vi "frontEnd.vi"(8 "error in (no error)":errorcluster, 11 "PixelflySettings in":refnum<class "PixelflySettings.lvclass">) -> (0 "error out":errorcluster, 3 "PixelflySettings out":refnum<class "PixelflySettings.lvclass">)   [LabVIEW 2009, in "Tools.lvlib" / "Settings.lvlib" / "PixelflySettings.lvclass"]
uses:
  PixelflySettings.lvclass
  PixelflySettings.lvclass/PixelflySettings.ctl
panel:
  out "Path":path
  in  "Mode":enum16{"Asynch Shutter", "Video"}(ring)=enum."Video"
  in  "Vertical Binning":enum16{"1", "2"}(ring)
  in  "Horizonatal Binning":enum16{"1", "2"}(ring)
  in  "image_number":i32 caption="Image Number"
  in  "Close":bool
  in  "Open":bool
  in  "Save":bool
  in  "Triggering":bool
  in  "gain":enum16{"Low", "High"}(ring) caption="Gain"
  in  "exposure":dbl(slide)=0.0064 min=1e-05 max=10.0 step=1e-05 scale=0.01..10.0 scale format="%^#_6g"
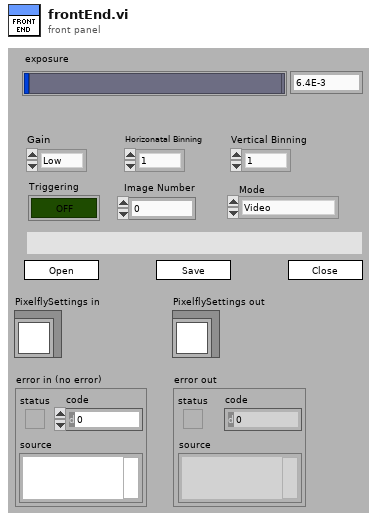
[diagram p1: front panel]
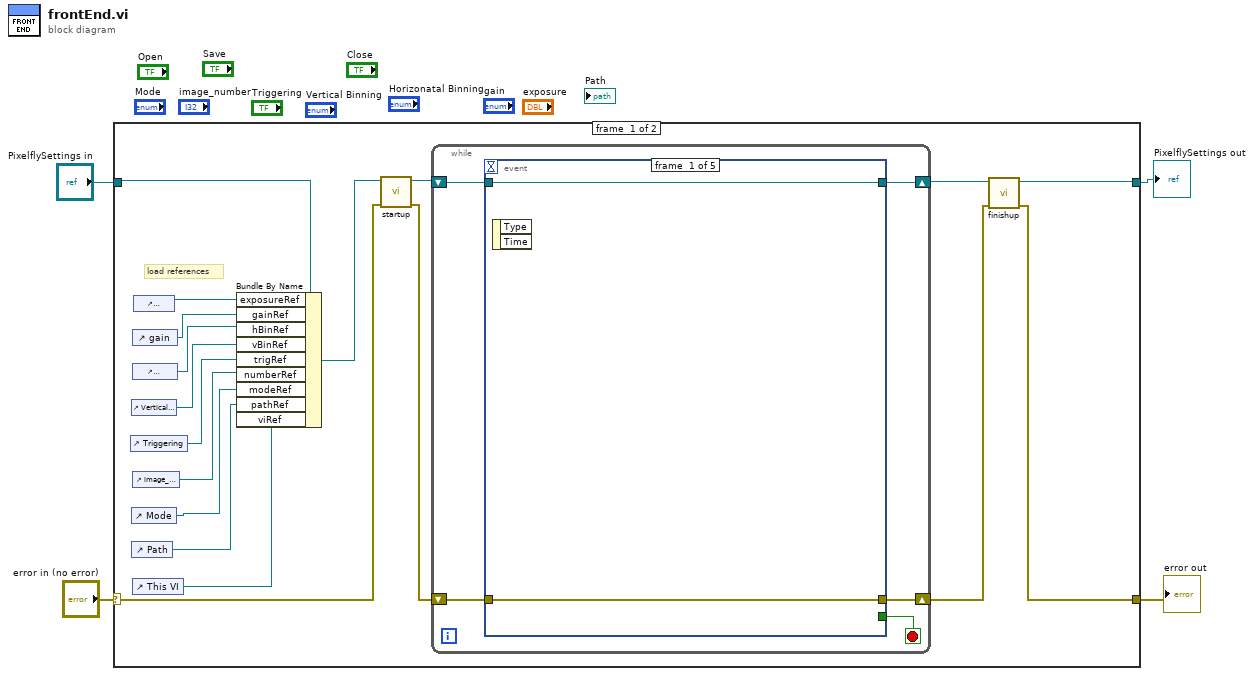
[diagram p0: block diagram]
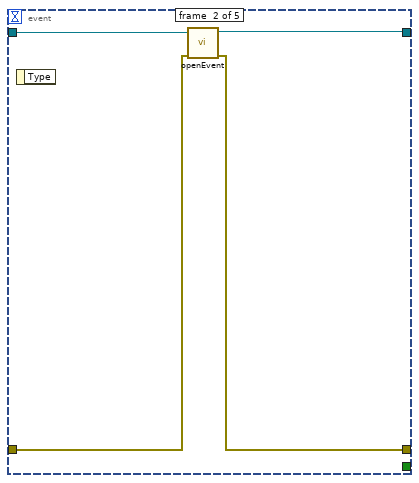
[diagram p2: hidden frame]
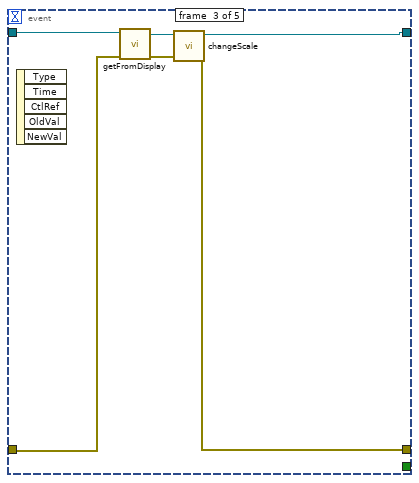
[diagram p3: hidden frame]
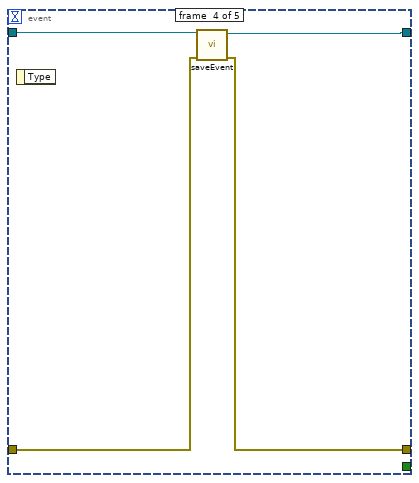
[diagram p4: hidden frame]
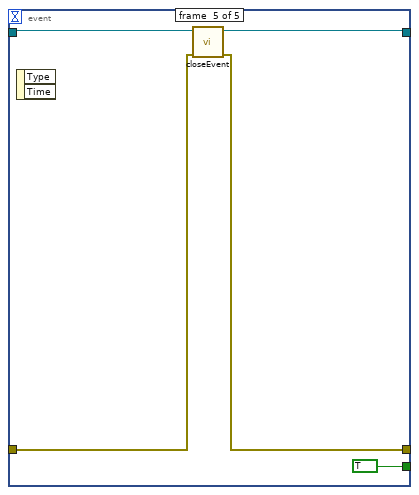
[diagram p5: hidden frame]
diagram:
  n1 = case shown="No Error" "error in (no error)" {
    selector: "error in (no error)" -> [w21 w49]
    tunnel: [w16 w49] -> w3
    tunnel: [w18 w50] -> w2
    tunnel: "PixelflySettings in" -> [w8 w50]
    frame #0 {
      # "load references"
      n2 = control-ref of="Triggering"() -> (w11:refnum<vi>)
      n3 = control-ref of="Vertical Binning"() -> (w12:refnum<vi>)
      n4 = control-ref of="Mode"() -> (w9:refnum<vi>)
      n5 = control-ref of="Path"() -> (w6:refnum<vi>)
      n6 = control-ref of="gain"() -> (w14:refnum<vi>)
      n7 = control-ref of="Horizonatal Binning"() -> (w13:refnum<vi>)
      n8 = control-ref of="image_number"() -> (w10:refnum<vi>)
      n9 = control-ref of="This VI"() -> (w5:refnum<vi>)
      n10 = control-ref of="exposure"() -> (w15:refnum<vi>)
      n11 = Bundle By Name(cluster=w8, "exposureRef"=w15, "gainRef"=w14, "hBinRef"=w13, "vBinRef"=w12, "trigRef"=w11, "numberRef"=w10, "modeRef"=w9, "pathRef"=w6, "viRef"=w5) -> (w7:refnum<class "PixelflySettings.lvclass">)
      n12 = call "startup.vi"("error in (no error)"=w21, "PixelflySettings in"=w7) -> ("error out"=w20:errorcluster, "PixelflySettings out"=w22:refnum<class "PixelflySettings.lvclass">)  [unwired: 8 in]
      n13 = while {
        shift-right: [w27] -> w19
        shift-left: w22 -> [w26]
        shift-right: [w25] -> w17
        shift-left: w20 -> [w24]
        stop <- w23 stop-if-true
        n14 = event shown="[4] \"Close\": Mouse Down;  Panel Close" {
          selector: _ -> [_ _ _ _ _]
          dyn-events: _ -> [_ _ _ _ _]
          timeout: _ -> [_ _ _ _ _]
          tunnel: [w29 w32 w39 w42 w46] -> w27
          tunnel: w26 -> [w29 w33 w36 w43 w47]
          tunnel: [w28 w30 w38 w40 w44] -> w25
          tunnel: w24 -> [w28 w31 w34 w41 w45]
          tunnel: [_ _ _ _ TRUE] -> w23
          event #0 {
            n15 = event-data() -> ()  [unwired: 1 in, 2 out]
          }
          event #1 {
            n16 = event-data() -> ()  [unwired: 1 in, 1 out]
            n17 = call "openEvent.vi"("error in (no error)"=w31, "PixelflySettings in"=w33) -> ("error out"=w30:errorcluster, "PixelflySettings out"=w32:refnum<class "PixelflySettings.lvclass">)  [unwired: 8 in]
          }
          event #2 {
            n18 = event-data() -> ()  [unwired: 1 in, 5 out]
            n19 = call "getFromDisplay.vi"("error in (no error)"=w34, "PixelflySettings in"=w36) -> ("error out"=w35:errorcluster, "PixelflySettings out"=w37:refnum<class "PixelflySettings.lvclass">)  [unwired: 8 in]
            n20 = call "changeScale.vi"("error in (no error)"=w35, "PixelflySettings in"=w37) -> ("error out"=w38:errorcluster, "PixelflySettings out"=w39:refnum<class "PixelflySettings.lvclass">)  [unwired: 8 in]
          }
          event #3 {
            n21 = event-data() -> ()  [unwired: 1 in, 1 out]
            n22 = call "saveEvent.vi"("error in (no error)"=w41, "PixelflySettings in"=w43) -> ("error out"=w40:errorcluster, "PixelflySettings out"=w42:refnum<class "PixelflySettings.lvclass">)  [unwired: 8 in]
          }
          event #4 {
            n23 = event-data() -> ()  [unwired: 1 in, 2 out]
            n24 = call "closeEvent.vi"("error in (no error)"=w45, "PixelflySettings in"=w47) -> ("error out"=w44:errorcluster, "PixelflySettings out"=w46:refnum<class "PixelflySettings.lvclass">)  [unwired: 8 in]
          }
        }
      }
      n25 = call "finishup.vi"("error in (no error)"=w17, "PixelflySettings in"=w19) -> ("error out"=w16:errorcluster, "PixelflySettings out"=w18:refnum<class "PixelflySettings.lvclass">)  [unwired: 8 in]
    }
    frame #1 {
    }
  }
  "error out" <- w3
  "PixelflySettings out" <- w2
